vi "JOG_Query.vi"(0 "System no.":i32=1 min=1 max=4 step=1, 2 "Axes to query":string[](array[string]), 3 "All axes?":bool, 4 "Axis identifier?":bool=TRUE, 5 "error in":errorcluster) -> (14 "JOG velocity":dbl[](array[numeric]) format="%.6f", 19 "error out":errorcluster)   [LabVIEW 2020]
doc: "Get the velocity and direction for motion caused by JOG."
panel:
  # "Get the velocity and direction for motion caused by JOG."
  # "If all axes: use"
  # "Query"
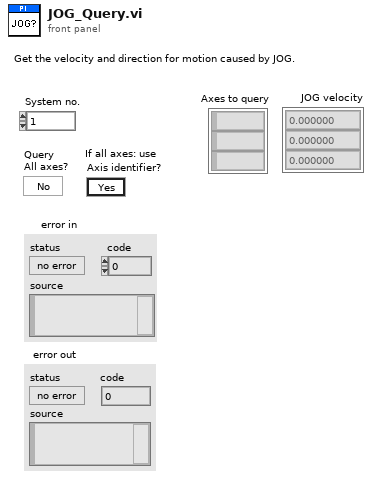
[diagram p1: front panel]
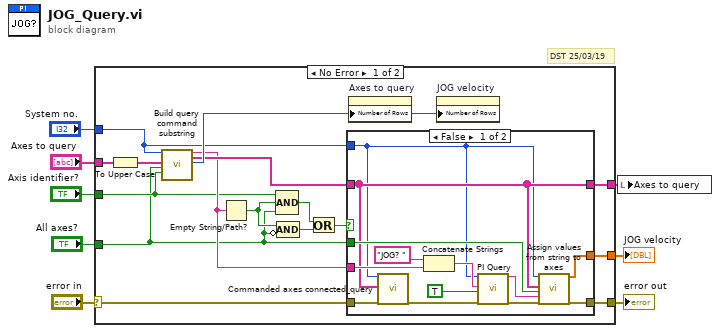
[diagram p0: block diagram]
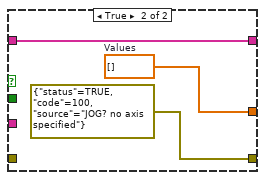
[diagram p2: hidden frame]
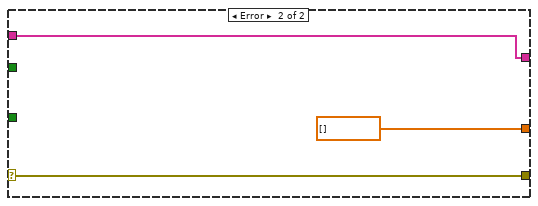
[diagram p3: hidden frame]
diagram:
  # "DST 25/03/19"
  n1 = case shown="No Error" "error in" {
    selector: "error in" -> [w13 w42]
    tunnel: [w24 dbl[] [] ("Values")] -> w8
    tunnel: "Axes to query" -> [w23 w41]
    tunnel: [w17 w42] -> w6
    tunnel: "System no." -> [w20 _]
    tunnel: [w14 w41] -> w4
    tunnel: "Axis identifier?" -> [w10 _]
    tunnel: "All axes?" -> [w9 _]
    frame No Error {
      n2 = To Upper Case(1:w23) -> (0:w22:string[])
      n3 = call "Build query command substring.vi"("System no."=w20, "Axes to query in"=w22, "Query\nAll axes?"=w9, "For all axes: use\nAxis identifier?"=w10) -> ("Command substring"=w12:string, "Axes to query out"=w15:string[], "Number of rows"=w21:u32)  [unwired: 2 in, 11 out]
      n4 = Empty String/Path?(string/path=w12) -> (empty?=w11:bool)
      n5 = Compound Arithmetic op=AND(w10, w11, w9) -> (w18:bool)
      n6 = Compound Arithmetic op=AND(w11, invert w9) -> (w19:bool)
      n7 = Or(x=w18, y=w19) -> (x .or. y?=w16:bool)
      n8 = case shown="False" w16 {
        tunnel: w12 -> [w29 _]
        tunnel: [w36 w39] -> w24
        tunnel: w20 -> [w27 _]
        tunnel: w15 -> [w28 w38]
        tunnel: w9 -> [w35 _]
        tunnel: [w34 errorcluster {"status"=TRUE, "code"=100, "source"="JOG? no axis specified"} ("error out")] -> w17
        tunnel: [w28 w38] -> w14
        tunnel: w13 -> [w25 _]
        frame False {
          n9 = call "Commanded axes connected_query.vi"("System no."=w27, "Commanded axes"=w28, "error in"=w25) -> ("error out"=w26:errorcluster)  [unwired: 1 in, 15 out]
          n10 = Concatenate Strings("JOG? ", w29) -> (w30:string)
          n11 = call "PI Query.vi"("System no."=w27, "String to send"=w30, "Attach termination char.?"=TRUE ("Attach Linefeed?"), "error in"=w26) -> ("String read"=w33:string, "error out"=w32:errorcluster)  [unwired: 3 in, 11 out]
          n12 = call "Assign values from string to axes.vi"("System no."=w27, "Queried axes"=w28, "All axes queried?"=w35, "Input String"=w33, "error in"=w32) -> ("Values"=w36:dbl[], "error out"=w34:errorcluster)  [unwired: 4 in, 9 out]
        }
        frame True {
          w39 = dbl[] []  # Values
        }
      }
      n13 = property on="Axes to query" class="Arr (strict)"("Number of Rows"=w21) -> ()  [unwired: 2 in, 2 out]
      n14 = property on="JOG velocity" class="Arr (strict)"("Number of Rows"=w21) -> ()  [unwired: 2 in, 2 out]
    }
    frame Error {
    }
  }
  "error out" <- w6
  "JOG velocity" <- w8
  n15 = local write "Axes to query"(w4) -> ()
